vi "ManageDAQ.vi"(8 "error in":errorcluster, 9 "StreamCluster_TypeDef":T1={"DAQ_Configs"=[], "CTR_Config"={"CTR refDes"="CTR001", "CTR IP Addr"="localhost"}, "Network_Configs"={"Buffer"=1, "ManagmentRate_Hz"=1000, "StreamRate_Hz"=10, "ConnectionHysterisis"=0, "LoggingRate_Hz"=10}, "ConfigXML_Checksum"=""}) -> (0 "error out":errorcluster, 1 "StreamCluster_TypeDef":T1={"DAQ_Configs"=[], "CTR_Config"={"CTR refDes"="CTR001", "CTR IP Addr"="localhost"}, "Network_Configs"={"Buffer"=1, "ManagmentRate_Hz"=1000, "StreamRate_Hz"=10, "ConnectionHysterisis"=0, "LoggingRate_Hz"=10}, "ConfigXML_Checksum"=""})   [LabVIEW 2024]
uses:
  Control/StreamCluster_TypeDef.ctl
  Control/streamIO_states.ctl
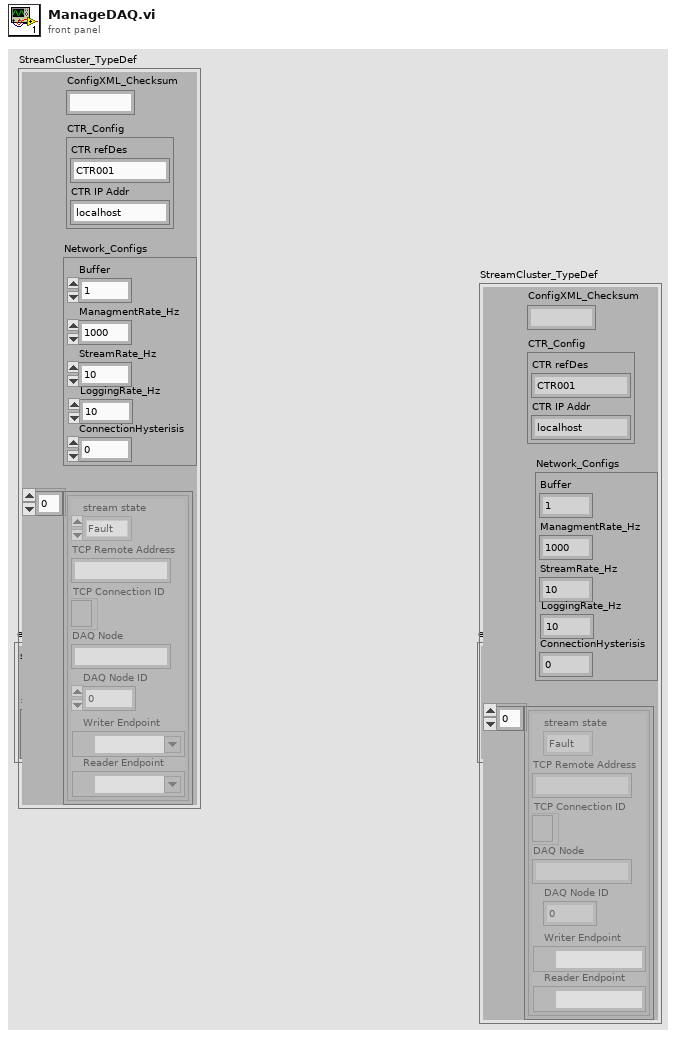
[diagram p1: front panel]
types:
  T1 = typedef "StreamCluster_TypeDef.ctl" = cluster{"DAQ_Configs":cluster{"stream state":T2, "TCP Remote Address":string, "TCP Connection ID":refnum<k5>, "DAQ Node":string, "DAQ Node ID":i32, "Writer Endpoint":refnum<k21>, "Reader Endpoint":refnum<k21>}[], "CTR_Config":cluster{"CTR refDes":string, "CTR IP Addr":string}, "Network_Configs":cluster{"Buffer":i32, "ManagmentRate_Hz":i32, "StreamRate_Hz":i32, "ConnectionHysterisis":i32, "LoggingRate_Hz":i32}, "ConfigXML_Checksum":string}
  T2 = typedef "streamIO_states.ctl" = enum16{"Fault", "Initialize", "Stream", "Close"}
  T3 = cluster{"stream state":T2, "TCP Remote Address":string, "TCP Connection ID":refnum<k5>, "DAQ Node":string, "DAQ Node ID":i32, "Writer Endpoint":refnum<k21>, "Reader Endpoint":refnum<k21>}[]
  T4 = cluster{"stream state":T2, "TCP Remote Address":string, "TCP Connection ID":refnum<k5>, "DAQ Node":string, "DAQ Node ID":i32, "Writer Endpoint":refnum<k21>, "Reader Endpoint":refnum<k21>}
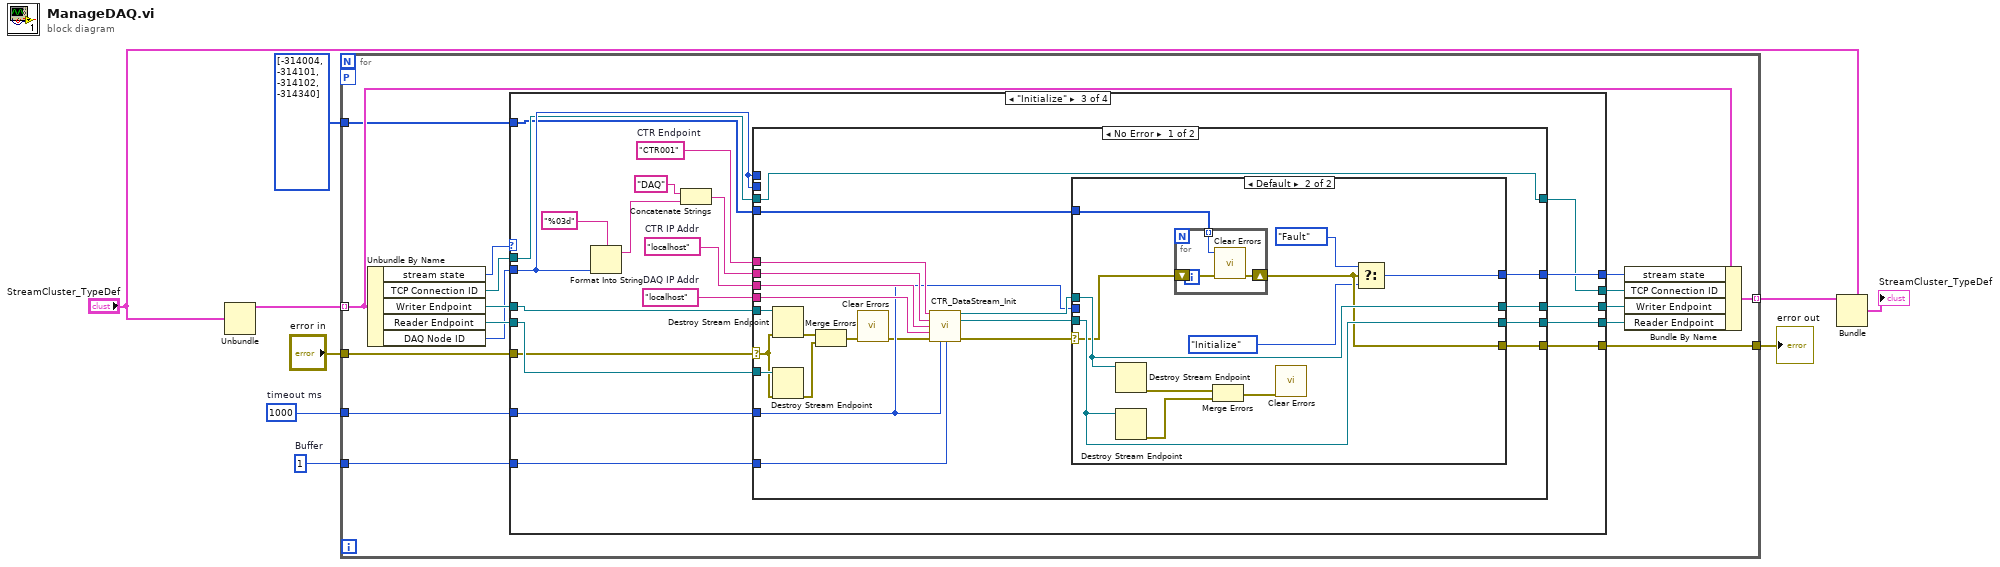
[diagram p0: block diagram]
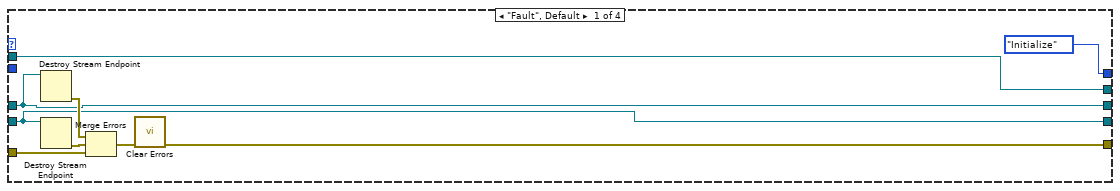
[diagram p2: hidden frame]
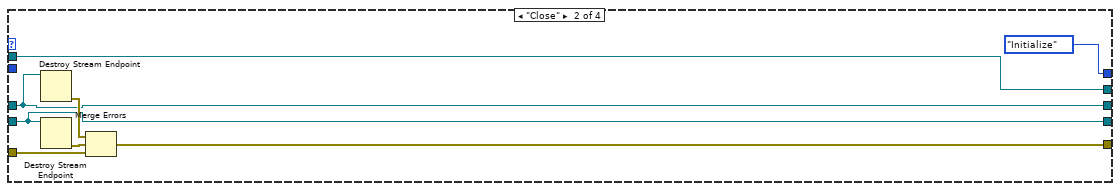
[diagram p3: hidden frame]
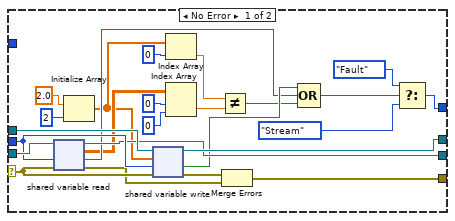
[diagram p4: hidden frame]
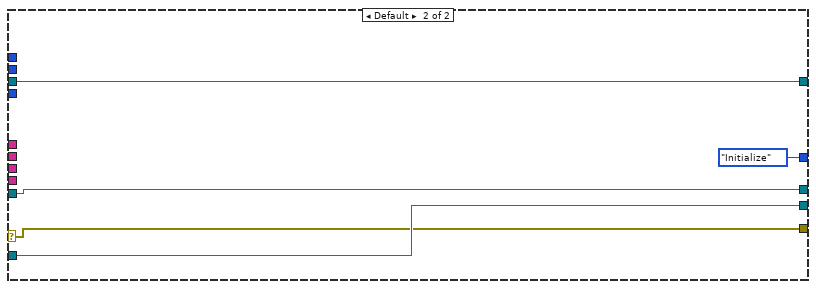
[diagram p5: hidden frame]
diagram:
  w7 = 1  # Buffer
  w8 = 1000  # timeout ms
  n1 = Unbundle("StreamCluster_TypeDef") -> ("DAQ_Configs"=w6:T3)  [unwired: 3 out]
  n2 = for {
    tunnel: "error in" -> [w16]
    tunnel: w8 -> [w14]
    tunnel: w7 -> [w25]
    tunnel: [w21] -> w5 mode=indexing
    tunnel: w6 -> [w20] mode=indexing
    workers-P: _ -> [_]
    tunnel: [w13] -> w2
    tunnel: i32[] [-314004, -314101, -314102, -314340] -> [w10]
    n3 = Unbundle By Name(w20) -> ("stream state"=w12:T2, "TCP Connection ID"=w11:refnum<k5>, "Writer Endpoint"=w23:refnum<k21>, "Reader Endpoint"=w22:refnum<k21>, "DAQ Node ID"=w19:i32)
    n4 = case shown="\"Initialize\"" w12 {
      selector: w12 -> [_ _ _ w133]
      tunnel: w25 -> [_ _ w62 _]
      tunnel: [streamIO_states."Initialize" ("stream state") streamIO_states."Initialize" ("stream state") w60 w133] -> w24
      tunnel: w23 -> [w28 w37 w59 w131]
      tunnel: w22 -> [w27 w36 w58 w130]
      tunnel: w19 -> [_ _ w50 _]
      tunnel: [w28 w37 w57 w131] -> w18
      tunnel: [w27 w36 w56 w130] -> w17
      tunnel: w16 -> [w32 w40 w44 w129]
      tunnel: [w33 w41 w55 w132] -> w15
      tunnel: w14 -> [_ _ w54 _]
      tunnel: [w26 w35 w52 w129] -> w13
      tunnel: w11 -> [w33 w41 w45 w132]
      tunnel: w10 -> [_ _ w43 _]
      frame "Fault", Default {
        n5 = Destroy Stream Endpoint(11:w28) -> (0:w29:errorcluster)  [unwired: 1 in]
        n6 = Destroy Stream Endpoint(11:w27) -> (0:w31:errorcluster)  [unwired: 1 in]
        n7 = Merge Errors(w29, w31, w32) -> (w30:errorcluster)
        n8 = call <vilib>:"Clear Errors.vi"("error in (no error)"=w30) -> ("error out"=w26:errorcluster)  [unwired: 5 in, 1 out]
      }
      frame "Close" {
        n9 = Destroy Stream Endpoint(11:w37) -> (0:w38:errorcluster)  [unwired: 1 in]
        n10 = Destroy Stream Endpoint(11:w36) -> (0:w39:errorcluster)  [unwired: 1 in]
        n11 = Merge Errors(w38, w39, w40) -> (w35:errorcluster)
      }
      frame "Initialize" {
        w46 = "localhost"  # DAQ IP Addr
        w61 = "localhost"  # CTR IP Addr
        w53 = "CTR001"  # CTR Endpoint
        n12 = Format Into String(format string="%03d", w50) -> (resulting string=w48:string)  [unwired: 2 in, 1 out]
        n13 = Concatenate Strings("DAQ" ("DAQ IR Addr"), w48) -> (w47:string)
        n14 = case shown="No Error" w44 {
          selector: w44 -> [w64 w124]
          tunnel: [w84 w124] -> w52
          tunnel: w47 -> [w78 _]
          tunnel: [w83 streamIO_states."Initialize" ("stream state")] -> w60
          tunnel: w61 -> [w82 _]
          tunnel: w53 -> [w81 _]
          tunnel: w50 -> [_ _]
          tunnel: w62 -> [w76 _]
          tunnel: w54 -> [w73 _]
          tunnel: w50 -> [_ _]
          tunnel: [w72 w127] -> w57
          tunnel: [w71 w126] -> w56
          tunnel: w59 -> [w66 w127]
          tunnel: w58 -> [w65 w126]
          tunnel: w45 -> [w80 w125]
          tunnel: [w80 w125] -> w55
          tunnel: w46 -> [w79 _]
          tunnel: w43 -> [w70 _]
          frame No Error {
            n15 = Destroy Stream Endpoint(8:w64, 11:w66) -> (0:w68:errorcluster)
            n16 = Destroy Stream Endpoint(8:w64, 11:w65) -> (0:w67:errorcluster)
            n17 = Merge Errors(w68, w67) -> (w69:errorcluster)
            n18 = call <vilib>:"Clear Errors.vi"("error in (no error)"=w69) -> ("error out"=w63:errorcluster)  [unwired: 5 in, 1 out]
            n19 = call "CTR_DataStream_Init.vi"("CTR Endpoint"=w81, "DAQ Endpoint"=w78, "CTR IP Addr"=w82, "DAQ IP Addr"=w79, "error in"=w63, "timeout ms"=w73, "Buffer"=w76) -> ("writer endpoint"=w75:refnum<k21>, "reader endpoint"=w74:refnum<k21>, "error out"=w77:errorcluster)  [unwired: 6 in]
            n20 = case shown="Default" w77 {
              selector: w77 -> [w107 w115]
              tunnel: [w103 w114] -> w84
              tunnel: [w85 w112] -> w83
              tunnel: w75 -> [w109 w117]
              tunnel: w74 -> [w108 w116]
              tunnel: w73 -> [w106 _]
              tunnel: [w105 w117] -> w72
              tunnel: [w104 w116] -> w71
              tunnel: w70 -> [_ w110]
              frame No Error {
                n21 = shared-variable-read(w108, w107, w106) -> (w104:refnum<k21>, w101:errorcluster, w99:bool, w97:dbl[][])
                n22 = Initialize Array(2.0 ("element"), 2 ("dimension size")) -> (w91:dbl[])
                n23 = shared-variable-write(w109, w107, w91, w106) -> (w105:refnum<k21>, w102:errorcluster, w100:bool)
                n24 = Index Array(array=w91, index=0) -> (element=w89:dbl)
                n25 = Index Array(array=w97, index (row)=0, index (col)=0) -> (element=w94:dbl)
                n26 = Not Equal?(x=w89, y=w94) -> (x != y?=w98:bool)
                n27 = Merge Errors(w102, w101) -> (w103:errorcluster)
                n28 = Compound Arithmetic op=OR(w100, w99, w98) -> (w88:bool)
                n29 = Select(t=streamIO_states."Fault" ("stream state"), s=w88, f=streamIO_states."Stream" ("stream state")) -> (s? t:f=w85:T2)
              }
              frame Default {
                n30 = Destroy Stream Endpoint(11:w117) -> (0:w119:errorcluster)  [unwired: 1 in]
                n31 = Destroy Stream Endpoint(11:w116) -> (0:w118:errorcluster)  [unwired: 1 in]
                n32 = for {
                  shift-right: [w122] -> w114
                  shift-left: w115 -> [w123]
                  tunnel: w110 -> [w121] mode=indexing
                  n33 = call <vilib>:"Clear Errors.vi"("error in (no error)"=w123, "specific error code to clear (0: all)"=w121) -> ("error out"=w122:errorcluster)  [unwired: 4 in, 1 out]
                }
                n34 = Merge Errors(w119, w118) -> (w120:errorcluster)
                n35 = call <vilib>:"Clear Errors.vi"("error in (no error)"=w120) -> ()  [unwired: 5 in, 2 out]
                n36 = Select(t=streamIO_states."Fault" ("stream state"), s=w114, f=streamIO_states."Initialize" ("stream state")) -> (s? t:f=w112:T2)
              }
            }
          }
          frame Default {
          }
        }
      }
      frame "Stream" {
      }
    }
    n37 = Bundle By Name(cluster=w20, "stream state"=w24, "TCP Connection ID"=w15, "Writer Endpoint"=w18, "Reader Endpoint"=w17) -> (w21:T4)
  }
  "error out" <- w2
  n38 = Bundle(cluster="StreamCluster_TypeDef", "DAQ_Configs"=w5) -> (→"StreamCluster_TypeDef":T1)  [unwired: 3 in]
